vi "Lab Panel V6.00.vi"() -> ()   [LabVIEW 2017] (continued)
                    n2215 = Multiply(x=w3882, y=w3876) -> (x*y=w3869:dbl)
                    n2216 = Multiply(x=w3881, y=w3875) -> (x*y=w3868:dbl)
                    n2217 = Multiply(x=w3880, y=w3874) -> (x*y=w3867:dbl)
                    n2218 = Multiply(x=w3879, y=w3873) -> (x*y=w3865:dbl)
                    n2219 = Multiply(x=w3878, y=w3872) -> (x*y=w3864:dbl)
                    n2220 = Multiply(x=w3877, y=w3871) -> (x*y=w3863:dbl)
                    n2221 = local read "SIG LAB02-1"() -> (w3870:T2)
                    n2222 = local read "SIG LAB02-2"() -> (w3866:T2)
                    n2223 = Bundle By Name(cluster=w3870, "AMPS"=w3869, "VOLTS"=w3868, "PF"=w3867) -> (w3862:T2)
                    n2224 = Bundle By Name(cluster=w3866, "AMPS"=w3865, "VOLTS"=w3864, "PF"=w3863) -> (w3861:T2)
                    n2225 = global write "Global display 1.vi" "SIG LAB02-1"(w3862) -> ()
                    n2226 = local write "SIG LAB02-2"(w3861) -> ()
                    n2227 = global write "Global display 1.vi" "SIG LAB02-2"(w3861) -> ()
                    n2228 = local write "SIG LAB02-1"(w3862) -> ()
                  }
                  frame #4 {
                    n2229 = Unbundle By Name(w3914) -> ("OFF amps"=w3910:dbl, "VOLTS"=w3909:dbl, "PF"=w3908:dbl, "OFF amps"=w3907:dbl, "VOLTS"=w3906:dbl, "PF"=w3905:dbl)
                    n2230 = case shown="True" w3913 {
                      tunnel: [w3915 w3916] -> w3911
                      tunnel: w3912 -> [_ w3916]
                      frame False {
                        n2231 = local read "CAL LAB03"() -> (w3915:T15)
                      }
                      frame True {
                      }
                    }
                    n2232 = Unbundle By Name(w3911) -> ("1  (A) cal"=w3904:dbl, "1 (V) cal"=w3903:dbl, "1 (PF) cal"=w3902:dbl, "2 (A) cal"=w3901:dbl, "2 (V) cal"=w3900:dbl, "2 (PF) cal"=w3899:dbl)  [unwired: 4 out]
                    n2233 = Multiply(x=w3910, y=w3904) -> (x*y=w3897:dbl)
                    n2234 = Multiply(x=w3909, y=w3903) -> (x*y=w3891:dbl)
                    n2235 = Multiply(x=w3908, y=w3902) -> (x*y=w3896:dbl)
                    n2236 = Multiply(x=w3907, y=w3901) -> (x*y=w3894:dbl)
                    n2237 = Multiply(x=w3906, y=w3900) -> (x*y=w3893:dbl)
                    n2238 = Multiply(x=w3905, y=w3899) -> (x*y=w3892:dbl)
                    n2239 = local read "SIG LAB03-1"() -> (w3898:T2)
                    n2240 = local read "SIG LAB03-2"() -> (w3895:T2)
                    n2241 = Bundle By Name(cluster=w3898, "AMPS"=w3897, "VOLTS"=w3891, "PF"=w3896) -> (w3890:T2)
                    n2242 = Bundle By Name(cluster=w3895, "AMPS"=w3894, "VOLTS"=w3893, "PF"=w3892) -> (w3889:T2)
                    n2243 = global write "Global display 1.vi" "SIG LAB03-1"(w3890) -> ()
                    n2244 = global write "Global display 1.vi" "SIG LAB03-2"(w3889) -> ()
                    n2245 = local write "SIG LAB03-2"(w3889) -> ()
                    n2246 = local write "SIG LAB03-1"(w3890) -> ()
                  }
                  frame #5 {
                    n2247 = case shown="False" w3941 {
                      tunnel: [w3943 w3944] -> w3939
                      tunnel: w3940 -> [_ w3944]
                      frame False {
                        n2248 = local read "CAL LAB04"() -> (w3943:T15)
                      }
                      frame True {
                      }
                    }
                    n2249 = Unbundle By Name(w3942) -> ("OFF amps"=w3938:dbl, "VOLTS"=w3937:dbl, "PF"=w3936:dbl, "OFF amps"=w3935:dbl, "VOLTS"=w3934:dbl, "PF"=w3933:dbl)
                    n2250 = Unbundle By Name(w3939) -> ("1  (A) cal"=w3932:dbl, "1 (V) cal"=w3931:dbl, "1 (PF) cal"=w3930:dbl, "2 (A) cal"=w3929:dbl, "2 (V) cal"=w3928:dbl, "2 (PF) cal"=w3927:dbl)  [unwired: 4 out]
                    n2251 = Multiply(x=w3938, y=w3932) -> (x*y=w3925:dbl)
                    n2252 = Multiply(x=w3937, y=w3931) -> (x*y=w3924:dbl)
                    n2253 = Multiply(x=w3936, y=w3930) -> (x*y=w3923:dbl)
                    n2254 = Multiply(x=w3935, y=w3929) -> (x*y=w3921:dbl)
                    n2255 = Multiply(x=w3934, y=w3928) -> (x*y=w3920:dbl)
                    n2256 = Multiply(x=w3933, y=w3927) -> (x*y=w3919:dbl)
                    n2257 = local read "SIG LAB04-1"() -> (w3926:T2)
                    n2258 = local read "SIG LAB04-2"() -> (w3922:T2)
                    n2259 = Bundle By Name(cluster=w3926, "AMPS"=w3925, "VOLTS"=w3924, "PF"=w3923) -> (w3918:T2)
                    n2260 = Bundle By Name(cluster=w3922, "AMPS"=w3921, "VOLTS"=w3920, "PF"=w3919) -> (w3917:T2)
                    n2261 = global write "Global display 1.vi" "SIG LAB04-2"(w3917) -> ()
                    n2262 = global write "Global display 1.vi" "SIG LAB04-1"(w3918) -> ()
                    n2263 = local write "SIG LAB04-2"(w3917) -> ()
                    n2264 = local write "SIG LAB04-1"(w3918) -> ()
                  }
                  frame #6 {
                    n2265 = Unbundle By Name(w3970) -> ("OFF amps"=w3966:dbl, "VOLTS"=w3947:dbl, "PF"=w3965:dbl, "OFF amps"=w3964:dbl, "VOLTS"=w3963:dbl, "PF"=w3962:dbl)
                    n2266 = case shown="False" w3969 {
                      tunnel: [w3971 w3972] -> w3967
                      tunnel: w3968 -> [_ w3972]
                      frame False {
                        n2267 = local read "CAL LAB05"() -> (w3971:T15)
                      }
                      frame True {
                      }
                    }
                    n2268 = Unbundle By Name(w3967) -> ("1  (A) cal"=w3961:dbl, "1 (V) cal"=w3960:dbl, "1 (PF) cal"=w3959:dbl, "2 (A) cal"=w3958:dbl, "2 (V) cal"=w3957:dbl, "2 (PF) cal"=w3956:dbl)  [unwired: 4 out]
                    n2269 = Multiply(x=w3966, y=w3961) -> (x*y=w3954:dbl)
                    n2270 = Multiply(x=w3947, y=w3960) -> (x*y=w3953:dbl)
                    n2271 = Multiply(x=w3965, y=w3959) -> (x*y=w3952:dbl)
                    n2272 = Multiply(x=w3964, y=w3958) -> (x*y=w3950:dbl)
                    n2273 = Multiply(x=w3963, y=w3957) -> (x*y=w3949:dbl)
                    n2274 = Multiply(x=w3962, y=w3956) -> (x*y=w3948:dbl)
                    n2275 = local read "SIG LAB05-1"() -> (w3955:T2)
                    n2276 = local read "SIG LAB05-2"() -> (w3951:T2)
                    n2277 = Bundle By Name(cluster=w3955, "AMPS"=w3954, "VOLTS"=w3953, "PF"=w3952) -> (w3946:T2)
                    n2278 = Bundle By Name(cluster=w3951, "AMPS"=w3950, "VOLTS"=w3949, "PF"=w3948) -> (w3945:T2)
                    n2279 = global write "Global display 1.vi" "SIG LAB05-1"(w3946) -> ()
                    n2280 = global write "Global display 1.vi" "SIG LAB05-2"(w3945) -> ()
                    n2281 = local write "SIG LAB05-2"(w3945) -> ()
                    n2282 = local write "SIG LAB05-1"(w3946) -> ()
                  }
                  frame #7 {
                    n2283 = case shown="False" w3973 {
                      tunnel: w3975 -> [w3980 _]
                      tunnel: w3974 -> [w3979 _]
                      frame False {
                        # "update ambient referance temperature"
                        n2284 = case shown="True" w3980 {
                          tunnel: [w3982 100.0] -> w3981
                          frame False {
                            n2285 = local read "TEMP REF cal"() -> (w3982:dbl)
                          }
                          frame True {
                          }
                        }
                        n2286 = disable-structure shown="Disabled" {
                          frame Disabled {
                            n2287 = local read "Temp read loop"() -> ()  [unwired: 1 out]
                          }
                          frame Enabled {
                          }
                        }
                        n2288 = Multiply(x=w3981, y=w3979) -> (x*y=w3978:dbl)
                        n2289 = Subtract(x=w3978, y=272) -> (x-y=w3976:dbl)
                        "Amb Tp" <- w3976
                        n2290 = local write "Ref deg C"(w3976) -> ()
                        "deg C (volts)" <- w3979
                      }
                      frame True {
                      }
                    }
                  }
                }
              }
            }
          }
          frame #14 {
            # "save test data to file during testing"
            n2291 = local read "on loops"() -> (w4003:dbl)
            n2292 = Get Date/Time In Seconds() -> (seconds since 1Jan1904=w3984:timestamp)
            "File Time Stamp" <- w3984
            n2293 = local read "jig cycle"() -> (w4000:dbl)
            n2294 = Format Date/Time String(time format string (%c)="%H:%M%:%S", seconds (now)=w3984) -> (date/time string=w3988:string)  [unwired: 1 in]
            n2295 = Add(x=w4003, y=4) -> (x+y=w4001:dbl)
            n2296 = Build Array(w3988) -> (w3987:string[])
            n2297 = Equal?(x=w4000, y=3) -> (x = y?=w3986:bool)
            n2298 = Equal?(x=w4000, y=w4001) -> (x = y?=w3985:bool)
            n2299 = stacked-sequence {
              tunnel: w3999 -> [w4009 _ _ _ _ _ _ _ _ _]
              tunnel: w3998 -> [_ w4085 _ _ _ _ _ _ _ _]
              tunnel: w3997 -> [_ _ w4165 _ _ _ _ _ _ _]
              tunnel: w3996 -> [_ _ _ w4245 _ _ _ _ _ _]
              tunnel: w3995 -> [_ _ _ _ w4325 _ _ _ _ _]
              tunnel: w3994 -> [_ _ _ _ _ w4405 _ _ _ _]
              tunnel: w3993 -> [_ _ _ _ _ _ w4485 _ _ _]
              tunnel: w3992 -> [_ _ _ _ _ _ _ w4565 _ _]
              tunnel: w3991 -> [_ _ _ _ _ _ _ _ w4645 _]
              tunnel: w3990 -> [_ _ _ _ _ _ _ _ _ w4725]
              tunnel: w3987 -> [w4008 w4089 w4169 w4249 w4329 w4409 w4489 w4569 w4649 w4729]
              tunnel: w3986 -> [w4007 w4088 w4168 w4248 w4328 w4408 w4488 w4568 w4648 w4728]
              tunnel: w3985 -> [w4006 w4087 w4167 w4247 w4327 w4407 w4487 w4567 w4647 w4727]
              tunnel: w3984 -> [w4005 w4086 w4166 w4246 w4326 w4406 w4486 w4566 w4646 w4726]
              frame #0 {
                n2300 = case shown="True" w4009 {
                  tunnel: w4008 -> [_ w4014]
                  tunnel: w4007 -> [_ w4013]
                  tunnel: w4006 -> [_ w4011]
                  tunnel: w4005 -> [_ w4010]
                  frame False {
                  }
                  frame True {
                    n2301 = local read "SIG LAB01-1"() -> (w4016:T2)
                    n2302 = local read "ON L01-1"() -> (w4012:cluster{"amps":dbl, "volts":dbl, "pf":dbl})
                    n2303 = local read "DISP LAB01-1"() -> (w4015:T4)
                    n2304 = Unbundle(w4016) -> ("AMPS"=w4022:dbl, "VOLTS"=w4020:dbl, "PF"=w4019:dbl, "Tmp Live"=w4018:dbl, "Tmp Neut"=w4021:dbl)
                    n2305 = Unbundle(w4015) -> ("CYCLE"=w4017:dbl)  [unwired: 2 out]
                    n2306 = stacked-sequence {
                      tunnel: w4022 -> [w4026 w4045]
                      tunnel: w4021 -> [_ w4044]
                      tunnel: w4020 -> [w4025 w4043]
                      tunnel: w4019 -> [w4024 w4042]
                      tunnel: w4018 -> [_ w4041]
                      tunnel: w4017 -> [_ w4040]
                      tunnel: w4014 -> [_ w4039]
                      tunnel: w4013 -> [w4027 _]
                      tunnel: w4012 -> [w4023 w4037]
                      tunnel: w4011 -> [_ w4038]
                      tunnel: w4010 -> [_ w4033]
                      frame #0 {
                        n2307 = case shown="True" w4027 {
                          tunnel: w4026 -> [_ w4032]
                          tunnel: w4025 -> [_ w4031]
                          tunnel: w4024 -> [_ w4030]
                          tunnel: w4023 -> [_ w4028]
                          frame False {
                          }
                          frame True {
                            n2308 = Bundle(cluster=w4028, "amps"=w4032, "volts"=w4031, "pf"=w4030) -> (w4029:cluster{"amps":dbl, "volts":dbl, "pf":dbl})
                            n2309 = local write "ON L01-1"(w4029) -> ()
                          }
                        }
                      }
                      frame #1 {
                        n2310 = Unbundle(w4037) -> ("amps"=w4036:dbl, "volts"=w4035:dbl, "pf"=w4034:dbl)
                        n2311 = case shown="True" w4038 {
                          tunnel: w4045 -> [_ w4046]
                          tunnel: w4044 -> [_ w4084]
                          tunnel: w4043 -> [_ _]
                          tunnel: w4042 -> [_ _]
                          tunnel: w4041 -> [_ w4083]
                          tunnel: w4040 -> [_ w4082]
                          tunnel: w4039 -> [_ w4050]
                          tunnel: w4036 -> [_ w4047]
                          tunnel: w4035 -> [_ w4079]
                          tunnel: w4034 -> [_ w4078]
                          tunnel: w4033 -> [_ w4048]
                          frame False {
                          }
                          frame True {
                            n2312 = local read "TDMS LAB01-1"() -> (w4081:refnum<k34>)
                            n2313 = Build Array(w4079) -> (w4075:dbl[])
                            n2314 = Build Array(w4078) -> (w4074:dbl[])
                            n2315 = Build Array(w4083) -> (w4073:dbl[])
                            n2316 = Build Array(w4084) -> (w4072:dbl[])
                            n2317 = Build Array(w4047) -> (w4077:dbl[])
                            n2318 = Build Array(w4046) -> (w4076:dbl[])
                            n2319 = Build Array(w4082) -> (w4071:dbl[])
                            n2320 = Build Array("AMPS ON", "AMPS OFF", "VOLTS", "PF", "TEMP Live", "TEMP Neut", "CYCLE") -> (w4055:string[])
                            n2321 = Bundle By Name("Y"=w4077, "t0"=w4048) -> (w4070:waveform(dbl))  [unwired: 1 in]
                            n2322 = Bundle By Name("Y"=w4076, "t0"=w4048) -> (w4069:waveform(dbl))  [unwired: 1 in]
                            n2323 = Bundle By Name("Y"=w4075, "t0"=w4048) -> (w4068:waveform(dbl))  [unwired: 1 in]
                            n2324 = Bundle By Name("Y"=w4074, "t0"=w4048) -> (w4067:waveform(dbl))  [unwired: 1 in]
                            n2325 = Bundle By Name("Y"=w4073, "t0"=w4048) -> (w4066:waveform(dbl))  [unwired: 1 in]
                            n2326 = Bundle By Name("Y"=w4072, "t0"=w4048) -> (w4065:waveform(dbl))  [unwired: 1 in]
                            n2327 = Bundle By Name("Y"=w4071, "t0"=w4048) -> (w4064:waveform(dbl))  [unwired: 1 in]
                            n2328 = Build Array(w4070, w4069, w4068, w4067, w4066, w4065, w4064) -> (w4063:waveform(dbl)[])
                            n2329 = TDMS Write(0:w4081, 5:"TEST VALUES", 7:w4055, 9:w4063) -> (4:w4054:refnum<k34>, 6:w4053:string, 15:w4052:errorcluster)  [unwired: 2 in, 1 out]
                            n2330 = TDMS Write(0:w4054, 5:w4053, 7:"TIME", 9:w4050, 11:w4052) -> (15:w4049:errorcluster)  [unwired: 1 in, 3 out]
                            n2331 = local write "data file error"(w4049) -> ()
                          }
                        }
                      }
                    }
                  }
                }
              }
              frame #1 {
                n2332 = case shown="True" w4085 {
                  tunnel: w4089 -> [_ w4094]
                  tunnel: w4088 -> [_ w4093]
                  tunnel: w4087 -> [_ w4091]
                  tunnel: w4086 -> [_ w4090]
                  frame False {
                  }
                  frame True {
                    n2333 = local read "DISP LAB01-2"() -> (w4095:T4)
                    n2334 = local read "SIG LAB01-2"() -> (w4096:T2)
                    n2335 = local read "ON L01-2"() -> (w4092:cluster{"amps":dbl, "volts":dbl, "pf":dbl})
                    n2336 = Unbundle(w4096) -> ("AMPS"=w4102:dbl, "VOLTS"=w4100:dbl, "PF"=w4099:dbl, "Tmp Live"=w4098:dbl, "Tmp Neut"=w4101:dbl)
                    n2337 = Unbundle(w4095) -> ("CYCLE"=w4097:dbl)  [unwired: 2 out]
                    n2338 = stacked-sequence {
                      tunnel: w4102 -> [w4106 w4125]
                      tunnel: w4101 -> [_ w4124]
                      tunnel: w4100 -> [w4105 w4123]
                      tunnel: w4099 -> [w4104 w4122]
                      tunnel: w4098 -> [_ w4121]
                      tunnel: w4097 -> [_ w4120]
                      tunnel: w4094 -> [_ w4119]
                      tunnel: w4093 -> [w4107 _]
                      tunnel: w4092 -> [w4103 w4117]
                      tunnel: w4091 -> [_ w4118]
                      tunnel: w4090 -> [_ w4113]
                      frame #0 {
                        n2339 = case shown="True" w4107 {
                          tunnel: w4106 -> [_ w4112]
                          tunnel: w4105 -> [_ w4111]
                          tunnel: w4104 -> [_ w4110]
                          tunnel: w4103 -> [_ w4108]
                          frame False {
                          }
                          frame True {
                            n2340 = Bundle(cluster=w4108, "amps"=w4112, "volts"=w4111, "pf"=w4110) -> (w4109:cluster{"amps":dbl, "volts":dbl, "pf":dbl})
                            n2341 = local write "ON L01-2"(w4109) -> ()
                          }
                        }
                      }
                      frame #1 {
                        n2342 = Unbundle(w4117) -> ("amps"=w4116:dbl, "volts"=w4115:dbl, "pf"=w4114:dbl)
                        n2343 = case shown="True" w4118 {
                          tunnel: w4125 -> [_ w4157]
                          tunnel: w4124 -> [_ w4164]
                          tunnel: w4123 -> [_ _]
                          tunnel: w4122 -> [_ _]
                          tunnel: w4121 -> [_ w4163]
                          tunnel: w4120 -> [_ w4162]
                          tunnel: w4119 -> [_ w4127]
                          tunnel: w4116 -> [_ w4159]
                          tunnel: w4115 -> [_ w4158]
                          tunnel: w4114 -> [_ w4156]
                          tunnel: w4113 -> [_ w4148]
                          frame False {
                          }
                          frame True {
                            n2344 = local read "TDMS LAB01-2"() -> (w4161:refnum<k34>)
                            n2345 = Build Array(w4158) -> (w4153:dbl[])
                            n2346 = Build Array(w4156) -> (w4152:dbl[])
                            n2347 = Build Array(w4163) -> (w4151:dbl[])
                            n2348 = Build Array(w4164) -> (w4150:dbl[])
                            n2349 = Build Array(w4159) -> (w4155:dbl[])
                            n2350 = Build Array(w4157) -> (w4154:dbl[])
                            n2351 = Build Array(w4162) -> (w4149:dbl[])
                            n2352 = Build Array("AMPS ON", "AMPS OFF", "VOLTS", "PF", "TEMP Live", "TEMP Neut", "CYCLE") -> (w4132:string[])
                            n2353 = Bundle By Name("Y"=w4155, "t0"=w4148) -> (w4147:waveform(dbl))  [unwired: 1 in]
                            n2354 = Bundle By Name("Y"=w4154, "t0"=w4148) -> (w4146:waveform(dbl))  [unwired: 1 in]
                            n2355 = Bundle By Name("Y"=w4153, "t0"=w4148) -> (w4145:waveform(dbl))  [unwired: 1 in]
                            n2356 = Bundle By Name("Y"=w4152, "t0"=w4148) -> (w4144:waveform(dbl))  [unwired: 1 in]
                            n2357 = Bundle By Name("Y"=w4151, "t0"=w4148) -> (w4143:waveform(dbl))  [unwired: 1 in]
                            n2358 = Bundle By Name("Y"=w4150, "t0"=w4148) -> (w4142:waveform(dbl))  [unwired: 1 in]
                            n2359 = Bundle By Name("Y"=w4149, "t0"=w4148) -> (w4141:waveform(dbl))  [unwired: 1 in]
                            n2360 = Build Array(w4147, w4146, w4145, w4144, w4143, w4142, w4141) -> (w4140:waveform(dbl)[])
                            n2361 = TDMS Write(0:w4161, 5:"TEST VALUES", 7:w4132, 9:w4140) -> (4:w4131:refnum<k34>, 6:w4130:string, 15:w4129:errorcluster)  [unwired: 2 in, 1 out]
                            n2362 = TDMS Write(0:w4131, 5:w4130, 7:"TIME", 9:w4127, 11:w4129) -> (15:w4126:errorcluster)  [unwired: 1 in, 3 out]
                            n2363 = local write "data file error"(w4126) -> ()
                          }
                        }
                      }
                    }
                  }
                }
              }
              frame #2 {
                n2364 = case shown="True" w4165 {
                  tunnel: w4169 -> [_ w4174]
                  tunnel: w4168 -> [_ w4173]
                  tunnel: w4167 -> [_ w4171]
                  tunnel: w4166 -> [_ w4170]
                  frame False {
                  }
                  frame True {
                    n2365 = local read "DISP LAB02-1"() -> (w4175:T4)
                    n2366 = local read "SIG LAB02-1"() -> (w4176:T2)
                    n2367 = local read "ON L02-1"() -> (w4172:cluster{"amps":dbl, "volts":dbl, "pf":dbl})
                    n2368 = Unbundle(w4176) -> ("AMPS"=w4182:dbl, "VOLTS"=w4180:dbl, "PF"=w4179:dbl, "Tmp Live"=w4178:dbl, "Tmp Neut"=w4181:dbl)
                    n2369 = Unbundle(w4175) -> ("CYCLE"=w4177:dbl)  [unwired: 2 out]
                    n2370 = stacked-sequence {
                      tunnel: w4182 -> [w4186 w4205]
                      tunnel: w4181 -> [_ w4204]
                      tunnel: w4180 -> [w4185 w4203]
                      tunnel: w4179 -> [w4184 w4202]
                      tunnel: w4178 -> [_ w4201]
                      tunnel: w4177 -> [_ w4200]
                      tunnel: w4174 -> [_ w4199]
                      tunnel: w4173 -> [w4187 _]
                      tunnel: w4172 -> [w4183 w4197]
                      tunnel: w4171 -> [_ w4198]
                      tunnel: w4170 -> [_ w4193]
                      frame #0 {
                        n2371 = case shown="True" w4187 {
                          tunnel: w4186 -> [_ w4192]
                          tunnel: w4185 -> [_ w4191]
                          tunnel: w4184 -> [_ w4190]
                          tunnel: w4183 -> [_ w4188]
                          frame False {
                          }
                          frame True {
                            n2372 = Bundle(cluster=w4188, "amps"=w4192, "volts"=w4191, "pf"=w4190) -> (w4189:cluster{"amps":dbl, "volts":dbl, "pf":dbl})
                            n2373 = local write "ON L02-1"(w4189) -> ()
                          }
                        }
                      }
                      frame #1 {
                        n2374 = Unbundle(w4197) -> ("amps"=w4196:dbl, "volts"=w4195:dbl, "pf"=w4194:dbl)
                        n2375 = case shown="True" w4198 {
                          tunnel: w4205 -> [_ w4237]
                          tunnel: w4204 -> [_ w4244]
                          tunnel: w4203 -> [_ _]
                          tunnel: w4202 -> [_ _]
                          tunnel: w4201 -> [_ w4243]
                          tunnel: w4200 -> [_ w4242]
                          tunnel: w4199 -> [_ w4207]
                          tunnel: w4196 -> [_ w4239]
                          tunnel: w4195 -> [_ w4238]
                          tunnel: w4194 -> [_ w4236]
                          tunnel: w4193 -> [_ w4228]
                          frame False {
                          }
                          frame True {
                            n2376 = local read "TDMS LAB02-1"() -> (w4241:refnum<k34>)
                            n2377 = Build Array(w4238) -> (w4233:dbl[])
                            n2378 = Build Array(w4236) -> (w4232:dbl[])
                            n2379 = Build Array(w4243) -> (w4231:dbl[])
                            n2380 = Build Array(w4244) -> (w4230:dbl[])
                            n2381 = Build Array(w4239) -> (w4235:dbl[])
                            n2382 = Build Array(w4237) -> (w4234:dbl[])
                            n2383 = Build Array(w4242) -> (w4229:dbl[])
                            n2384 = Build Array("AMPS ON", "AMPS OFF", "VOLTS", "PF", "TEMP Live", "TEMP Neut", "CYCLE") -> (w4212:string[])
                            n2385 = Bundle By Name("Y"=w4235, "t0"=w4228) -> (w4227:waveform(dbl))  [unwired: 1 in]
                            n2386 = Bundle By Name("Y"=w4234, "t0"=w4228) -> (w4226:waveform(dbl))  [unwired: 1 in]
                            n2387 = Bundle By Name("Y"=w4233, "t0"=w4228) -> (w4225:waveform(dbl))  [unwired: 1 in]
                            n2388 = Bundle By Name("Y"=w4232, "t0"=w4228) -> (w4224:waveform(dbl))  [unwired: 1 in]
                            n2389 = Bundle By Name("Y"=w4231, "t0"=w4228) -> (w4223:waveform(dbl))  [unwired: 1 in]
                            n2390 = Bundle By Name("Y"=w4230, "t0"=w4228) -> (w4222:waveform(dbl))  [unwired: 1 in]
                            n2391 = Bundle By Name("Y"=w4229, "t0"=w4228) -> (w4221:waveform(dbl))  [unwired: 1 in]
                            n2392 = Build Array(w4227, w4226, w4225, w4224, w4223, w4222, w4221) -> (w4220:waveform(dbl)[])
                            n2393 = TDMS Write(0:w4241, 5:"TEST VALUES", 7:w4212, 9:w4220) -> (4:w4211:refnum<k34>, 6:w4210:string, 15:w4209:errorcluster)  [unwired: 2 in, 1 out]
                            n2394 = TDMS Write(0:w4211, 5:w4210, 7:"TIME", 9:w4207, 11:w4209) -> (15:w4206:errorcluster)  [unwired: 1 in, 3 out]
                            n2395 = local write "data file error"(w4206) -> ()
                          }
                        }
                      }
                    }
                  }
                }
              }
              frame #3 {
                n2396 = case shown="True" w4245 {
                  tunnel: w4249 -> [_ w4254]
                  tunnel: w4248 -> [_ w4253]
                  tunnel: w4247 -> [_ w4251]
                  tunnel: w4246 -> [_ w4250]
                  frame False {
                  }
                  frame True {
                    n2397 = local read "DISP LAB02-2"() -> (w4255:T4)
                    n2398 = local read "SIG LAB02-2"() -> (w4256:T2)
                    n2399 = local read "ON L02-2"() -> (w4252:cluster{"amps":dbl, "volts":dbl, "pf":dbl})
                    n2400 = Unbundle(w4256) -> ("AMPS"=w4262:dbl, "VOLTS"=w4260:dbl, "PF"=w4259:dbl, "Tmp Live"=w4258:dbl, "Tmp Neut"=w4261:dbl)
                    n2401 = Unbundle(w4255) -> ("CYCLE"=w4257:dbl)  [unwired: 2 out]
                    n2402 = stacked-sequence {
                      tunnel: w4262 -> [w4266 w4285]
                      tunnel: w4261 -> [_ w4284]
                      tunnel: w4260 -> [w4265 w4283]
                      tunnel: w4259 -> [w4264 w4282]
                      tunnel: w4258 -> [_ w4281]
                      tunnel: w4257 -> [_ w4280]
                      tunnel: w4254 -> [_ w4279]
                      tunnel: w4253 -> [w4267 _]
                      tunnel: w4252 -> [w4263 w4277]
                      tunnel: w4251 -> [_ w4278]
                      tunnel: w4250 -> [_ w4273]
                      frame #0 {
                        n2403 = case shown="True" w4267 {
                          tunnel: w4266 -> [_ w4272]
                          tunnel: w4265 -> [_ w4271]
                          tunnel: w4264 -> [_ w4270]
                          tunnel: w4263 -> [_ w4268]
                          frame False {
                          }
                          frame True {
                            n2404 = Bundle(cluster=w4268, "amps"=w4272, "volts"=w4271, "pf"=w4270) -> (w4269:cluster{"amps":dbl, "volts":dbl, "pf":dbl})
                            n2405 = local write "ON L02-2"(w4269) -> ()
                          }
                        }
                      }
                      frame #1 {
                        n2406 = Unbundle(w4277) -> ("amps"=w4276:dbl, "volts"=w4275:dbl, "pf"=w4274:dbl)
                        n2407 = case shown="True" w4278 {
                          tunnel: w4285 -> [_ w4317]
                          tunnel: w4284 -> [_ w4324]
                          tunnel: w4283 -> [_ _]
                          tunnel: w4282 -> [_ _]
                          tunnel: w4281 -> [_ w4323]
                          tunnel: w4280 -> [_ w4322]
                          tunnel: w4279 -> [_ w4287]
                          tunnel: w4276 -> [_ w4319]
                          tunnel: w4275 -> [_ w4318]
                          tunnel: w4274 -> [_ w4316]
                          tunnel: w4273 -> [_ w4308]
                          frame False {
                          }
                          frame True {
                            n2408 = local read "TDMS LAB02-2"() -> (w4321:refnum<k34>)
                            n2409 = Build Array(w4318) -> (w4313:dbl[])
                            n2410 = Build Array(w4316) -> (w4312:dbl[])
                            n2411 = Build Array(w4323) -> (w4311:dbl[])
                            n2412 = Build Array(w4324) -> (w4310:dbl[])
                            n2413 = Build Array(w4319) -> (w4315:dbl[])
                            n2414 = Build Array(w4317) -> (w4314:dbl[])
                            n2415 = Build Array(w4322) -> (w4309:dbl[])
                            n2416 = Build Array("AMPS ON", "AMPS OFF", "VOLTS", "PF", "TEMP Live", "TEMP Neut", "CYCLE") -> (w4292:string[])
                            n2417 = Bundle By Name("Y"=w4315, "t0"=w4308) -> (w4307:waveform(dbl))  [unwired: 1 in]
                            n2418 = Bundle By Name("Y"=w4314, "t0"=w4308) -> (w4306:waveform(dbl))  [unwired: 1 in]
                            n2419 = Bundle By Name("Y"=w4313, "t0"=w4308) -> (w4305:waveform(dbl))  [unwired: 1 in]
                            n2420 = Bundle By Name("Y"=w4312, "t0"=w4308) -> (w4304:waveform(dbl))  [unwired: 1 in]
                            n2421 = Bundle By Name("Y"=w4311, "t0"=w4308) -> (w4303:waveform(dbl))  [unwired: 1 in]
                            n2422 = Bundle By Name("Y"=w4310, "t0"=w4308) -> (w4302:waveform(dbl))  [unwired: 1 in]
                            n2423 = Bundle By Name("Y"=w4309, "t0"=w4308) -> (w4301:waveform(dbl))  [unwired: 1 in]
                            n2424 = Build Array(w4307, w4306, w4305, w4304, w4303, w4302, w4301) -> (w4300:waveform(dbl)[])
                            n2425 = TDMS Write(0:w4321, 5:"TEST VALUES", 7:w4292, 9:w4300) -> (4:w4291:refnum<k34>, 6:w4290:string, 15:w4289:errorcluster)  [unwired: 2 in, 1 out]
                            n2426 = TDMS Write(0:w4291, 5:w4290, 7:"TIME", 9:w4287, 11:w4289) -> (15:w4286:errorcluster)  [unwired: 1 in, 3 out]
                            n2427 = local write "data file error"(w4286) -> ()
                          }
                        }
                      }
                    }
                  }
                }
              }
              frame #4 {
                n2428 = case shown="True" w4325 {
                  tunnel: w4329 -> [_ w4334]
                  tunnel: w4328 -> [_ w4333]
                  tunnel: w4327 -> [_ w4331]
                  tunnel: w4326 -> [_ w4330]
                  frame False {
                  }
                  frame True {
                    n2429 = local read "DISP LAB03-1"() -> (w4335:T4)
                    n2430 = local read "SIG LAB03-1"() -> (w4336:T2)
                    n2431 = local read "ON L03-1"() -> (w4332:cluster{"amps":dbl, "volts":dbl, "pf":dbl})
                    n2432 = Unbundle(w4336) -> ("AMPS"=w4342:dbl, "VOLTS"=w4340:dbl, "PF"=w4339:dbl, "Tmp Live"=w4338:dbl, "Tmp Neut"=w4341:dbl)
                    n2433 = Unbundle(w4335) -> ("CYCLE"=w4337:dbl)  [unwired: 2 out]
                    n2434 = stacked-sequence {
                      tunnel: w4342 -> [w4346 w4365]
                      tunnel: w4341 -> [_ w4364]
                      tunnel: w4340 -> [w4345 w4363]
                      tunnel: w4339 -> [w4344 w4362]
                      tunnel: w4338 -> [_ w4361]
                      tunnel: w4337 -> [_ w4360]
                      tunnel: w4334 -> [_ w4359]
                      tunnel: w4333 -> [w4347 _]
                      tunnel: w4332 -> [w4343 w4357]
                      tunnel: w4331 -> [_ w4358]
                      tunnel: w4330 -> [_ w4353]
                      frame #0 {
                        n2435 = case shown="True" w4347 {
                          tunnel: w4346 -> [_ w4352]
                          tunnel: w4345 -> [_ w4351]
                          tunnel: w4344 -> [_ w4350]
                          tunnel: w4343 -> [_ w4348]
                          frame False {
                          }
                          frame True {
                            n2436 = Bundle(cluster=w4348, "amps"=w4352, "volts"=w4351, "pf"=w4350) -> (w4349:cluster{"amps":dbl, "volts":dbl, "pf":dbl})
                            n2437 = local write "ON L03-1"(w4349) -> ()
                          }
                        }
                      }
                      frame #1 {
                        n2438 = Unbundle(w4357) -> ("amps"=w4356:dbl, "volts"=w4355:dbl, "pf"=w4354:dbl)
                        n2439 = case shown="True" w4358 {
                          tunnel: w4365 -> [_ w4397]
                          tunnel: w4364 -> [_ w4404]
                          tunnel: w4363 -> [_ _]
                          tunnel: w4362 -> [_ _]
                          tunnel: w4361 -> [_ w4403]
                          tunnel: w4360 -> [_ w4402]
                          tunnel: w4359 -> [_ w4367]
                          tunnel: w4356 -> [_ w4399]
                          tunnel: w4355 -> [_ w4398]
                          tunnel: w4354 -> [_ w4396]
                          tunnel: w4353 -> [_ w4388]
                          frame False {
                          }
                          frame True {
                            n2440 = local read "TDMS LAB03-1"() -> (w4401:refnum<k34>)
                            n2441 = Build Array(w4398) -> (w4393:dbl[])
                            n2442 = Build Array(w4396) -> (w4392:dbl[])
                            n2443 = Build Array(w4403) -> (w4391:dbl[])
                            n2444 = Build Array(w4404) -> (w4390:dbl[])
                            n2445 = Build Array(w4399) -> (w4395:dbl[])
                            n2446 = Build Array(w4397) -> (w4394:dbl[])
                            n2447 = Build Array(w4402) -> (w4389:dbl[])
                            n2448 = Build Array("AMPS ON", "AMPS OFF", "VOLTS", "PF", "TEMP Live", "TEMP Neut", "CYCLE") -> (w4372:string[])
                            n2449 = Bundle By Name("Y"=w4395, "t0"=w4388) -> (w4387:waveform(dbl))  [unwired: 1 in]
                            n2450 = Bundle By Name("Y"=w4394, "t0"=w4388) -> (w4386:waveform(dbl))  [unwired: 1 in]
                            n2451 = Bundle By Name("Y"=w4393, "t0"=w4388) -> (w4385:waveform(dbl))  [unwired: 1 in]
                            n2452 = Bundle By Name("Y"=w4392, "t0"=w4388) -> (w4384:waveform(dbl))  [unwired: 1 in]
                            n2453 = Bundle By Name("Y"=w4391, "t0"=w4388) -> (w4383:waveform(dbl))  [unwired: 1 in]
                            n2454 = Bundle By Name("Y"=w4390, "t0"=w4388) -> (w4382:waveform(dbl))  [unwired: 1 in]
                            n2455 = Bundle By Name("Y"=w4389, "t0"=w4388) -> (w4381:waveform(dbl))  [unwired: 1 in]
                            n2456 = Build Array(w4387, w4386, w4385, w4384, w4383, w4382, w4381) -> (w4380:waveform(dbl)[])
                            n2457 = TDMS Write(0:w4401, 5:"TEST VALUES", 7:w4372, 9:w4380) -> (4:w4371:refnum<k34>, 6:w4370:string, 15:w4369:errorcluster)  [unwired: 2 in, 1 out]
                            n2458 = TDMS Write(0:w4371, 5:w4370, 7:"TIME", 9:w4367, 11:w4369) -> (15:w4366:errorcluster)  [unwired: 1 in, 3 out]
                            n2459 = local write "data file error"(w4366) -> ()
                          }
                        }
                      }
                    }
                  }
                }
              }
              frame #5 {
                n2460 = case shown="True" w4405 {
                  tunnel: w4409 -> [_ w4414]
                  tunnel: w4408 -> [_ w4413]
                  tunnel: w4407 -> [_ w4411]
                  tunnel: w4406 -> [_ w4410]
                  frame False {
                  }
                  frame True {
                    n2461 = local read "DISP LAB03-2"() -> (w4415:T4)
                    n2462 = local read "SIG LAB03-2"() -> (w4416:T2)
                    n2463 = local read "ON L03-2"() -> (w4412:cluster{"amps":dbl, "volts":dbl, "pf":dbl})
                    n2464 = Unbundle(w4416) -> ("AMPS"=w4422:dbl, "VOLTS"=w4420:dbl, "PF"=w4419:dbl, "Tmp Live"=w4418:dbl, "Tmp Neut"=w4421:dbl)
                    n2465 = Unbundle(w4415) -> ("CYCLE"=w4417:dbl)  [unwired: 2 out]
                    n2466 = stacked-sequence {
                      tunnel: w4422 -> [w4426 w4445]
                      tunnel: w4421 -> [_ w4444]
                      tunnel: w4420 -> [w4425 w4443]
                      tunnel: w4419 -> [w4424 w4442]
                      tunnel: w4418 -> [_ w4441]
                      tunnel: w4417 -> [_ w4440]
                      tunnel: w4414 -> [_ w4439]
                      tunnel: w4413 -> [w4427 _]
                      tunnel: w4412 -> [w4423 w4437]
                      tunnel: w4411 -> [_ w4438]
                      tunnel: w4410 -> [_ w4433]
                      frame #0 {
                        n2467 = case shown="True" w4427 {
                          tunnel: w4426 -> [_ w4432]
                          tunnel: w4425 -> [_ w4431]
                          tunnel: w4424 -> [_ w4430]
                          tunnel: w4423 -> [_ w4428]
                          frame False {
                          }
                          frame True {
                            n2468 = Bundle(cluster=w4428, "amps"=w4432, "volts"=w4431, "pf"=w4430) -> (w4429:cluster{"amps":dbl, "volts":dbl, "pf":dbl})
                            n2469 = local write "ON L03-2"(w4429) -> ()
                          }
                        }
                      }
                      frame #1 {
                        n2470 = Unbundle(w4437) -> ("amps"=w4436:dbl, "volts"=w4435:dbl, "pf"=w4434:dbl)
                        n2471 = case shown="True" w4438 {
                          tunnel: w4445 -> [_ w4477]
                          tunnel: w4444 -> [_ w4484]
                          tunnel: w4443 -> [_ _]
                          tunnel: w4442 -> [_ _]
                          tunnel: w4441 -> [_ w4483]
                          tunnel: w4440 -> [_ w4482]
                          tunnel: w4439 -> [_ w4447]
                          tunnel: w4436 -> [_ w4479]
                          tunnel: w4435 -> [_ w4478]
                          tunnel: w4434 -> [_ w4476]
                          tunnel: w4433 -> [_ w4468]
                          frame False {
                          }
                          frame True {
                            n2472 = local read "TDMS LAB03-2"() -> (w4481:refnum<k34>)
                            n2473 = Build Array(w4478) -> (w4473:dbl[])
                            n2474 = Build Array(w4476) -> (w4472:dbl[])
                            n2475 = Build Array(w4483) -> (w4471:dbl[])
                            n2476 = Build Array(w4484) -> (w4470:dbl[])
                            n2477 = Build Array(w4479) -> (w4475:dbl[])
                            n2478 = Build Array(w4477) -> (w4474:dbl[])
                            n2479 = Build Array(w4482) -> (w4469:dbl[])
                            n2480 = Build Array("AMPS ON", "AMPS OFF", "VOLTS", "PF", "TEMP Live", "TEMP Neut", "CYCLE") -> (w4452:string[])
                            n2481 = Bundle By Name("Y"=w4475, "t0"=w4468) -> (w4467:waveform(dbl))  [unwired: 1 in]
                            n2482 = Bundle By Name("Y"=w4474, "t0"=w4468) -> (w4466:waveform(dbl))  [unwired: 1 in]
                            n2483 = Bundle By Name("Y"=w4473, "t0"=w4468) -> (w4465:waveform(dbl))  [unwired: 1 in]
                            n2484 = Bundle By Name("Y"=w4472, "t0"=w4468) -> (w4464:waveform(dbl))  [unwired: 1 in]
                            n2485 = Bundle By Name("Y"=w4471, "t0"=w4468) -> (w4463:waveform(dbl))  [unwired: 1 in]
                            n2486 = Bundle By Name("Y"=w4470, "t0"=w4468) -> (w4462:waveform(dbl))  [unwired: 1 in]
                            n2487 = Bundle By Name("Y"=w4469, "t0"=w4468) -> (w4461:waveform(dbl))  [unwired: 1 in]
                            n2488 = Build Array(w4467, w4466, w4465, w4464, w4463, w4462, w4461) -> (w4460:waveform(dbl)[])
                            n2489 = TDMS Write(0:w4481, 5:"TEST VALUES", 7:w4452, 9:w4460) -> (4:w4451:refnum<k34>, 6:w4450:string, 15:w4449:errorcluster)  [unwired: 2 in, 1 out]
                            n2490 = TDMS Write(0:w4451, 5:w4450, 7:"TIME", 9:w4447, 11:w4449) -> (15:w4446:errorcluster)  [unwired: 1 in, 3 out]
                            n2491 = local write "data file error"(w4446) -> ()
                          }
                        }
                      }
                    }
                  }
                }
              }
              frame #6 {
                n2492 = case shown="True" w4485 {
                  tunnel: w4489 -> [_ w4494]
                  tunnel: w4488 -> [_ w4493]
                  tunnel: w4487 -> [_ w4491]
                  tunnel: w4486 -> [_ w4490]
                  frame False {
                  }
                  frame True {
                    n2493 = local read "DISP LAB04-1"() -> (w4495:T4)
                    n2494 = local read "SIG LAB04-1"() -> (w4496:T2)
                    n2495 = local read "ON L04-1"() -> (w4492:cluster{"amps":dbl, "volts":dbl, "pf":dbl})
                    n2496 = Unbundle(w4496) -> ("AMPS"=w4502:dbl, "VOLTS"=w4500:dbl, "PF"=w4499:dbl, "Tmp Live"=w4498:dbl, "Tmp Neut"=w4501:dbl)
                    n2497 = Unbundle(w4495) -> ("CYCLE"=w4497:dbl)  [unwired: 2 out]
                    n2498 = stacked-sequence {
                      tunnel: w4502 -> [w4506 w4525]
                      tunnel: w4501 -> [_ w4524]
                      tunnel: w4500 -> [w4505 w4523]
                      tunnel: w4499 -> [w4504 w4522]
                      tunnel: w4498 -> [_ w4521]
                      tunnel: w4497 -> [_ w4520]
                      tunnel: w4494 -> [_ w4519]
                      tunnel: w4493 -> [w4507 _]
                      tunnel: w4492 -> [w4503 w4517]
                      tunnel: w4491 -> [_ w4518]
                      tunnel: w4490 -> [_ w4513]
                      frame #0 {
                        n2499 = case shown="True" w4507 {
                          tunnel: w4506 -> [_ w4512]
                          tunnel: w4505 -> [_ w4511]
                          tunnel: w4504 -> [_ w4510]
                          tunnel: w4503 -> [_ w4508]
                          frame False {
                          }
                          frame True {
                            n2500 = Bundle(cluster=w4508, "amps"=w4512, "volts"=w4511, "pf"=w4510) -> (w4509:cluster{"amps":dbl, "volts":dbl, "pf":dbl})
                            n2501 = local write "ON L04-1"(w4509) -> ()
                          }
                        }
                      }
                      frame #1 {
                        n2502 = Unbundle(w4517) -> ("amps"=w4516:dbl, "volts"=w4515:dbl, "pf"=w4514:dbl)
                        n2503 = case shown="True" w4518 {
                          tunnel: w4525 -> [_ w4557]
                          tunnel: w4524 -> [_ w4564]
                          tunnel: w4523 -> [_ _]
                          tunnel: w4522 -> [_ _]
                          tunnel: w4521 -> [_ w4563]
                          tunnel: w4520 -> [_ w4562]
                          tunnel: w4519 -> [_ w4527]
                          tunnel: w4516 -> [_ w4559]
                          tunnel: w4515 -> [_ w4558]
                          tunnel: w4514 -> [_ w4556]
                          tunnel: w4513 -> [_ w4548]
                          frame False {
                          }
                          frame True {
                            n2504 = local read "TDMS LAB04-1"() -> (w4561:refnum<k34>)
                            n2505 = Build Array(w4558) -> (w4553:dbl[])
                            n2506 = Build Array(w4556) -> (w4552:dbl[])
                            n2507 = Build Array(w4563) -> (w4551:dbl[])
                            n2508 = Build Array(w4564) -> (w4550:dbl[])
                            n2509 = Build Array(w4559) -> (w4555:dbl[])
                            n2510 = Build Array(w4557) -> (w4554:dbl[])
                            n2511 = Build Array(w4562) -> (w4549:dbl[])
                            n2512 = Build Array("AMPS ON", "AMPS OFF", "VOLTS", "PF", "TEMP Live", "TEMP Neut", "CYCLE") -> (w4532:string[])
                            n2513 = Bundle By Name("Y"=w4555, "t0"=w4548) -> (w4547:waveform(dbl))  [unwired: 1 in]
                            n2514 = Bundle By Name("Y"=w4554, "t0"=w4548) -> (w4546:waveform(dbl))  [unwired: 1 in]
                            n2515 = Bundle By Name("Y"=w4553, "t0"=w4548) -> (w4545:waveform(dbl))  [unwired: 1 in]
                            n2516 = Bundle By Name("Y"=w4552, "t0"=w4548) -> (w4544:waveform(dbl))  [unwired: 1 in]
                            n2517 = Bundle By Name("Y"=w4551, "t0"=w4548) -> (w4543:waveform(dbl))  [unwired: 1 in]
                            n2518 = Bundle By Name("Y"=w4550, "t0"=w4548) -> (w4542:waveform(dbl))  [unwired: 1 in]
                            n2519 = Bundle By Name("Y"=w4549, "t0"=w4548) -> (w4541:waveform(dbl))  [unwired: 1 in]
                            n2520 = Build Array(w4547, w4546, w4545, w4544, w4543, w4542, w4541) -> (w4540:waveform(dbl)[])
                            n2521 = TDMS Write(0:w4561, 5:"TEST VALUES", 7:w4532, 9:w4540) -> (4:w4531:refnum<k34>, 6:w4530:string, 15:w4529:errorcluster)  [unwired: 2 in, 1 out]
                            n2522 = TDMS Write(0:w4531, 5:w4530, 7:"TIME", 9:w4527, 11:w4529) -> (15:w4526:errorcluster)  [unwired: 1 in, 3 out]
                            n2523 = local write "data file error"(w4526) -> ()
                          }
                        }
                      }
                    }
                  }
                }
              }
              frame #7 {
                n2524 = case shown="True" w4565 {
                  tunnel: w4569 -> [_ w4574]
                  tunnel: w4568 -> [_ w4573]
                  tunnel: w4567 -> [_ w4571]
                  tunnel: w4566 -> [_ w4570]
                  frame False {
                  }
                  frame True {
                    n2525 = local read "DISP LAB04-2"() -> (w4575:T4)
                    n2526 = local read "SIG LAB04-2"() -> (w4576:T2)
                    n2527 = local read "ON L04-2"() -> (w4572:cluster{"amps":dbl, "volts":dbl, "pf":dbl})
                    n2528 = Unbundle(w4576) -> ("AMPS"=w4582:dbl, "VOLTS"=w4580:dbl, "PF"=w4579:dbl, "Tmp Live"=w4578:dbl, "Tmp Neut"=w4581:dbl)
                    n2529 = Unbundle(w4575) -> ("CYCLE"=w4577:dbl)  [unwired: 2 out]
                    n2530 = stacked-sequence {
                      tunnel: w4582 -> [w4586 w4605]
                      tunnel: w4581 -> [_ w4604]
                      tunnel: w4580 -> [w4585 w4603]
                      tunnel: w4579 -> [w4584 w4602]
                      tunnel: w4578 -> [_ w4601]
                      tunnel: w4577 -> [_ w4600]
                      tunnel: w4574 -> [_ w4599]
                      tunnel: w4573 -> [w4587 _]
                      tunnel: w4572 -> [w4583 w4597]
                      tunnel: w4571 -> [_ w4598]
                      tunnel: w4570 -> [_ w4593]
                      frame #0 {
                        n2531 = case shown="True" w4587 {
                          tunnel: w4586 -> [_ w4592]
                          tunnel: w4585 -> [_ w4591]
                          tunnel: w4584 -> [_ w4590]
                          tunnel: w4583 -> [_ w4588]
                          frame False {
                          }
                          frame True {
                            n2532 = Bundle(cluster=w4588, "amps"=w4592, "volts"=w4591, "pf"=w4590) -> (w4589:cluster{"amps":dbl, "volts":dbl, "pf":dbl})
                            n2533 = local write "ON L04-2"(w4589) -> ()
                          }
                        }
                      }
                      frame #1 {
                        n2534 = Unbundle(w4597) -> ("amps"=w4596:dbl, "volts"=w4595:dbl, "pf"=w4594:dbl)
                        n2535 = case shown="True" w4598 {
                          tunnel: w4605 -> [_ w4637]
                          tunnel: w4604 -> [_ w4644]
                          tunnel: w4603 -> [_ _]
                          tunnel: w4602 -> [_ _]
                          tunnel: w4601 -> [_ w4643]
                          tunnel: w4600 -> [_ w4642]
                          tunnel: w4599 -> [_ w4607]
                          tunnel: w4596 -> [_ w4639]
                          tunnel: w4595 -> [_ w4638]
                          tunnel: w4594 -> [_ w4636]
                          tunnel: w4593 -> [_ w4628]
                          frame False {
                          }
                          frame True {
                            n2536 = local read "TDMS LAB04-2"() -> (w4641:refnum<k34>)
                            n2537 = Build Array(w4638) -> (w4633:dbl[])
                            n2538 = Build Array(w4636) -> (w4632:dbl[])
                            n2539 = Build Array(w4643) -> (w4631:dbl[])
